vi "TestCOMPortConnectionOpen.vi"() -> ()   [LabVIEW 2020]
uses:
  StageSelector--Enum.ctl
  <vilib>/Galil/resources/gclib32/gclib32.lvlib
panel:
  out "Stage Position":string
  out "error out":errorcluster
  in  "error IO":errorcluster
  in  "IPAddress\\COM":string="COM1 -b 19200"
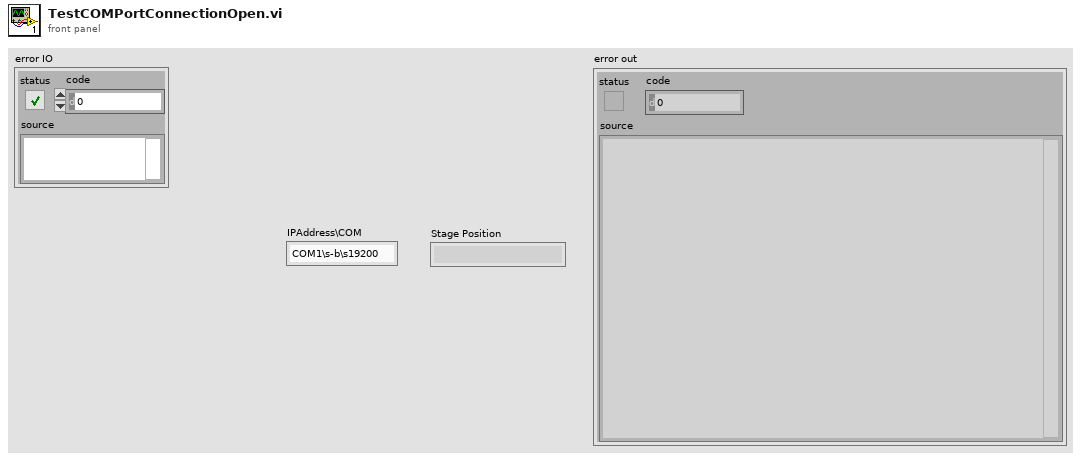
[diagram p1: front panel]
types:
  T1 = typedef "StageSelector--Enum.ctl" = enum16{"A", "B", "C", "D"}
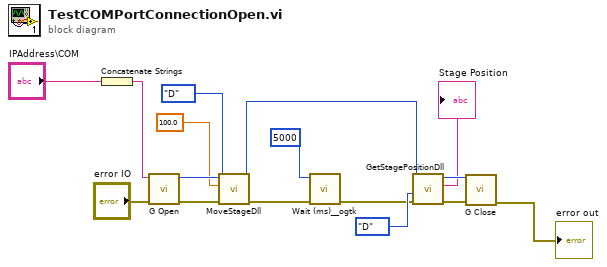
[diagram p0: block diagram]
diagram:
  n1 = Concatenate Strings("IPAddress\\COM") -> (w10:string)
  n2 = call <vilib>:"G Open.vi"("error in (no error)"="error IO", "address"=w10) -> ("error out"=w7:errorcluster, "g out"=w9:u32)  [unwired: 7 in]
  n3 = call "MoveStageDll.vi"("error in"=w7, "Stage"=StageSelector--Enum."D", "Z.pos"=100.0, "DevRefIn"=w9) -> ("error out"=w6:errorcluster, "DevRefOut"=w8:u32)  [unwired: 5 in, 1 out]
  n4 = call <userlib>:"Wait (ms)__ogtk.vi"("error in (no error)"=w6, "milliseconds to wait"=u32 5000) -> ("error out"=w2:errorcluster)  [unwired: 8 in, 1 out]
  n5 = call "GetStagePositionDll.vi"("error in"=w2, "Stage"=StageSelector--Enum."D", "DevRefIn"=w8) -> ("error out"=w14:errorcluster, "Stage Position"=→"Stage Position":string, "DevRefOut"=w13:u32)  [unwired: 6 in]
  n6 = call <vilib>:"G Close.vi"("error in (no error)"=w14, "g"=w13) -> ("error out"=→"error out":errorcluster)  [unwired: 9 in]
